vi "Set message.vi"(10 "WampMessage JSON":refnum<class "WampMessage JSON.lvclass">, 11 "AbortHandler JSON in":refnum<class "AbortHandler JSON.lvclass">) -> (3 "AbortHandler JSON out":refnum<class "AbortHandler JSON.lvclass">)   [LabVIEW 2020, in "wamplv.lvlib" / "AbortHandler JSON.lvclass"]
uses:
  AbortHandler JSON.lvclass
  AbortHandler JSON.lvclass/AbortHandler JSON.ctl
  SerialisedMessages/JSONMessage/WampMessage JSON.lvclass
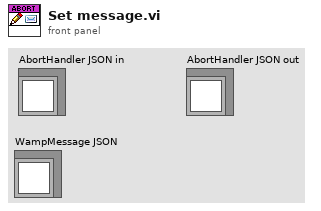
[diagram p1: front panel]
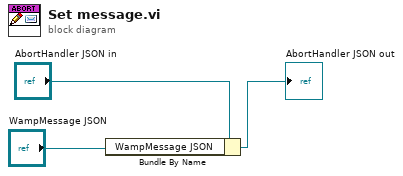
[diagram p0: block diagram]
diagram:
  n1 = Bundle By Name(cluster="AbortHandler JSON in", "WampMessage JSON"="WampMessage JSON") -> (→"AbortHandler JSON out":refnum<class "AbortHandler JSON.lvclass">)
